vi "transTime.vi"(1 "Channel":T2, 2 "subPacket":T1) -> (0 "delay":dbl)   [LabVIEW 2014]
uses:
  <vilib>/gmath/statdist.llb/Exp Random.vi
  <vilib>/gmath/NI_Gmath.lvlib
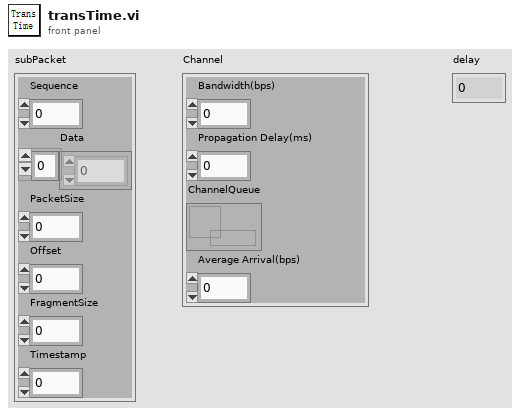
[diagram p1: front panel]
types:
  T1 = cluster{"Sequence":i32, "Data":u8[], "PacketSize":i32, "Offset":i32, "FragmentSize":i32, "Timestamp":i32}
  T2 = cluster{"Bandwidth(bps)":i32, "Propagation Delay(ms)":i32, "ChannelQueue":refnum<queue>, "Average Arrival(bps)":dbl}
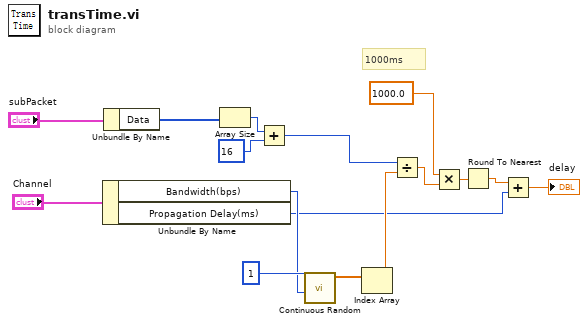
[diagram p0: block diagram]
diagram:
  # "1000ms"
  n1 = Unbundle By Name("Channel") -> ("Bandwidth(bps)"=w8:i32, "Propagation Delay(ms)"=w2:i32)
  n2 = Unbundle By Name("subPacket") -> ("Data"=w15:u8[])
  n3 = Array Size(array=w15) -> (size(s)=w14:i32)
  n4 = Add(x=w14, y=16) -> (x+y=w12:i32)
  n5 = call-poly <vilib>:"Continuous Random.vi"("b"=w8, "samples"=1) -> ("exp random data"=w10:dbl[])  [unwired: 8 in, 1 out]
  n6 = Index Array(array=w10) -> (element=w9:dbl)  [unwired: 1 in]
  n7 = Divide(x=w12, y=w9) -> (x/y=w5:dbl)
  n8 = Multiply(x=1000.0 ("y"), y=w5) -> (x*y=w4:dbl)
  n9 = Round To Nearest(number=w4) -> (nearest integer value=w3:dbl)
  n10 = Add(x=w3, y=w2) -> (x+y=→"delay":dbl)
